vi "Get Structure Key Hex.vi"(1 "Struct Options":T1, 2 "# Struct Elements":u8) -> (7 "Key":string)   [LabVIEW 2020, in "CBOR.lvlib"]
doc: "Get Structure key string based on the option selected."
uses:
  CBOR.lvlib
  Controls/Structure Options.ctl
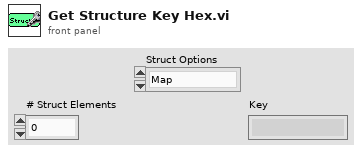
[diagram p1: front panel]
types:
  T1 = typedef "CBOR.lvlib/Structure Options.ctl" = enum16{"Map", "Text", "Array", "Integer", "Float"}
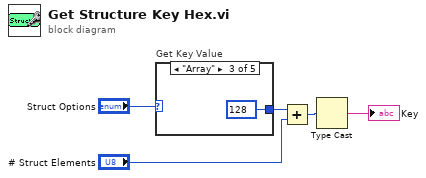
[diagram p0: block diagram]
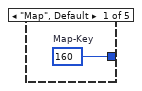
[diagram p2: hidden frame]
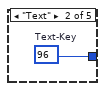
[diagram p3: hidden frame]
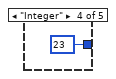
[diagram p4: hidden frame]
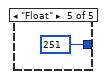
[diagram p5: hidden frame]
diagram:
  n1 = case "Get Key Value" shown="\"Array\"" "Struct Options" {
    tunnel: [w6 w7 u8 128 ("Text-Key") u8 23 ("Text-Key") u8 251 ("Text-Key")] -> w4
    frame "Map", Default {
      w6 = u8 160  # Map-Key
    }
    frame "Text" {
      w7 = u8 96  # Text-Key
    }
    frame "Array" {
    }
    frame "Integer" {
    }
    frame "Float" {
    }
  }
  n2 = Add(x=w4, y="# Struct Elements") -> (x+y=w2:u8)
  n3 = Type Cast(x=w2) -> (*(type *) &x=→"Key":string)  [unwired: 1 in]
